vi "find_token.vi"(3 "tokens":string[](array[string])=["[", "]", "{", "}"], 5 "string in":string) -> (0 "found token":string, 1 "string before token":string, 2 "string after token":string)   [LabVIEW 2011]
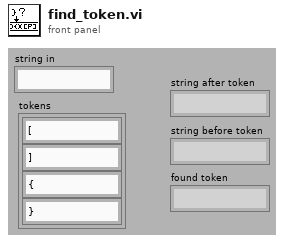
[diagram p1: front panel]
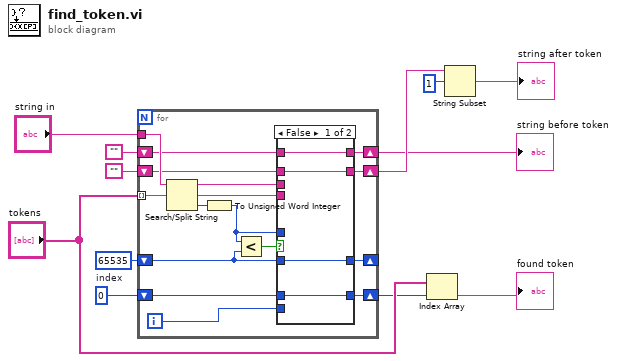
[diagram p0: block diagram]
diagram:
  w3 = u16 0  # index
  n1 = for {
    tunnel: "tokens" -> [w28] mode=indexing
    tunnel: "string in" -> [w27]
    shift-right: [w24] -> _
    shift-left: u16 65535 -> [w23]
    shift-right: [w21] -> w1
    shift-left: "" -> [w20]
    shift-right: [w18] -> w5
    shift-left: "" -> [w17]
    shift-right: [w14] -> w2
    shift-left: w3 -> [w15]
    i -> [w13]
    n2 = Search/Split String(string=w27, search string/char (-)=w28) -> (substring before match=w19:string, match + rest of string=w16:string, offset of match=w26:i32)  [unwired: 1 in]
    n3 = To Unsigned Word Integer(number=w26) -> (unsigned 16bit integer=w22:u16)
    n4 = Less?(x=w22, y=w23) -> (x < y?=w25:bool)
    n5 = case shown="False" w25 {
      tunnel: [w32 w36] -> w24
      tunnel: w23 -> [w32 _]
      tunnel: w22 -> [_ w36]
      tunnel: [w31 w35] -> w21
      tunnel: w20 -> [w31 _]
      tunnel: w19 -> [_ w35]
      tunnel: [w30 w34] -> w18
      tunnel: w17 -> [w30 _]
      tunnel: w16 -> [_ w34]
      tunnel: w15 -> [w29 _]
      tunnel: [w29 w33] -> w14
      tunnel: w13 -> [_ w33]
      frame False {
      }
      frame True {
      }
    }
  }
  "string before token" <- w1
  n6 = Index Array(array="tokens", index=w2) -> (element=→"found token":string)
  n7 = String Subset(string=w5, offset (0)=1) -> (substring=→"string after token":string)  [unwired: 1 in]
